vi "write_data_with_TCP.vi"(8 "error_in":errorcluster, 10 "data_in":dbl[](array[numeric]), 11 "TCP_ref_in":refnum<k5>) -> (0 "error_out":errorcluster, 3 "TCP_ref_out":refnum<k5>)   [LabVIEW 2020]
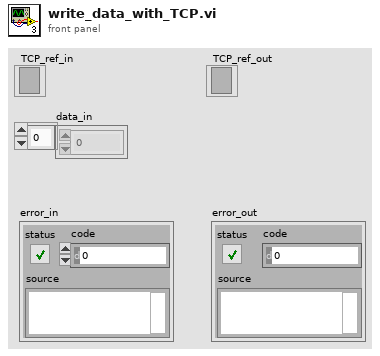
[diagram p1: front panel]
types:
  T1 = enum16{"big-endian, network order", "native, host order", "little-endian"}
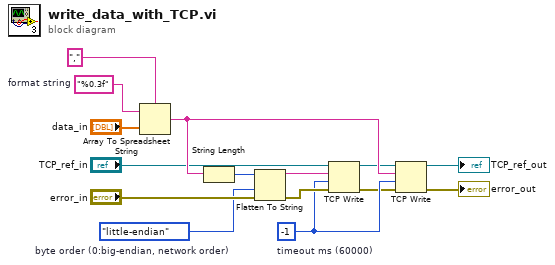
[diagram p0: block diagram]
diagram:
  w10 = -1  # timeout ms (60000)
  w11 = T1."little-endian"  # byte order (0:big-endian, network order)
  w3 = "%0.3f"  # format string
  n1 = Array To Spreadsheet String(delimiter (Tab)=",", array="data_in", 3:w3) -> (spreadsheet string=w13:string)
  n2 = String Length(string=w13) -> (length=w1:i32)
  n3 = Flatten To String(anything=w1, byte order (0:big-endian, network order)=w11, error in (no error)="error_in") -> (data string=w12:string, error out=w15:errorcluster)  [unwired: 1 in, 1 out]
  n4 = TCP Write(connection ID="TCP_ref_in", data in=w12, error in (no error)=w15, 9:w10) -> (connection ID out=w8:refnum<k5>, error out=w9:errorcluster)  [unwired: 1 out]
  n5 = TCP Write(connection ID=w8, data in=w13, error in (no error)=w9, 9:w10) -> (connection ID out=→"TCP_ref_out":refnum<k5>, error out=→"error_out":errorcluster)  [unwired: 1 out]
